vi "PH_SHS_Analysis_Statistician.PC Set Sample Length.vi"(0 "i ref in":refnum<vi>, 2 "Sample Length":i32, 5 "error IO":errorcluster) -> (14 "i ref out":refnum<vi>, 19 "error out":errorcluster)   [LabVIEW 2014, in "PH_SHS_Analysis_Statistician.lvlib"]
uses:
  PH_SHS_Analysis_Statistician.lvlib
  PH_Common/PH_Common.lvlib
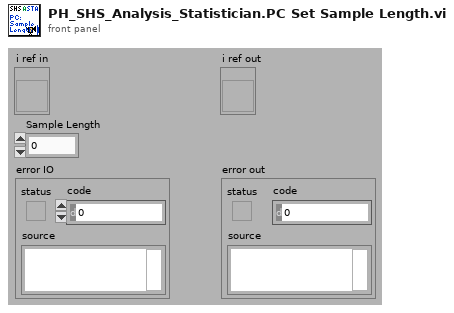
[diagram p1: front panel]
types:
  T1 = typedef "PH_SHS_Analysis_Statistician.lvlib/PH_SHS_Analysis_Statistician.i attribute.ctl" = cluster{"GUI Refs ":cluster{"Status":refnum<vi>, "Result Graph":refnum<vi>, "Mean Data 1":refnum<vi>, "Std Dev Data 1":refnum<vi>, "Mean Data 2":refnum<vi>, "Std Dev Data 2":refnum<vi>, "Mean Data 3":refnum<vi>, "Std Dev Data 3":refnum<vi>, "Dummy Mean":refnum<vi>, "Dummy Std Dev":refnum<vi>, "Export Data":refnum<vi>, "Data 1":refnum<vi>, "Data 2":refnum<vi>, "Data 3":refnum<vi>, "Stat or Trend":refnum<vi>, "Delete":refnum<vi>, "Analyzer":refnum<vi>, "Current Zernike Coefficients":refnum<vi>, "PtV [Lambda]":refnum<vi>, "sample length":refnum<vi>}, "Analyzer":string, "Stat or Trend":bool, "Data 1":i16, "Data 2":i16, "Data 3":i16, "Data":T2[], "sample length":i32, "Datasets strored":i32, "Dataarray Size":i32}
  T2 = typedef "PH_SHS_Analysis.lvlib/PH_SHS_Analysis.Zernike Dataset.ctl" = cluster{"State":T3, "Time Stamp":timestamp, "PtV [lambda]":dbl, "Zernicke Coefficients":T4}
  T3 = typedef "PH_StatusHandler.lvlib/PH_StatusHandler.Status.ctl" = i16
  T4 = typedef "PH_SHS_Analysis.lvlib/PH_SHS_Analysis.Zernike Coefficients.ctl" = cluster{"Tilt x":dbl, "Tilt y":dbl, "Defocus":dbl, "Astig 0°":dbl, "Astig 45°":dbl, "Coma x":dbl, "Coma y":dbl, "Spherical":dbl, "Trefoil 0°":dbl, "Trefoil 30°":dbl, "2nd Astig 0°":dbl, "2nd Astig 45°":dbl, "2nd Coma x":dbl, "2nd Coma y":dbl, "2nd Spherical":dbl}
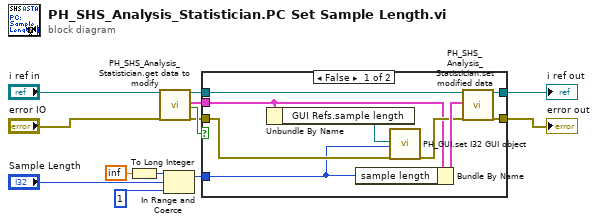
[diagram p0: block diagram]
diagram:
  n1 = To Long Integer(number=inf) -> (32bit integer=w2:i32)
  n2 = call "PH_SHS_Analysis_Statistician.get data to modify.vi"("i ref in"="i ref in", "error in (no error)"="error IO") -> ("i ref out"=w7:refnum<vi>, "i attribute"=w12:T1, "timed out"=w11:bool, "error out"=w9:errorcluster)  [unwired: 14 in]
  n3 = In Range and Coerce(upper limit=w2, x="Sample Length", lower limit=1) -> (coerced(x)=w4:i32)  [unwired: 1 out]
  n4 = case shown="False" w11 {
    tunnel: w7 -> [w22 w24]
    tunnel: [w21 w24] -> w8
    tunnel: w9 -> [w20 w23]
    tunnel: [w19 w23] -> w10
    tunnel: w12 -> [w15 _]
    tunnel: w4 -> [w16 _]
    frame False {
      n5 = Unbundle By Name(w15) -> ("GUI Refs.sample length"=w14:refnum<vi>)
      n6 = Bundle By Name(cluster=w15, "sample length"=w16) -> (w18:T1)
      n7 = call "PH_GUI.set I32 GUI object.vi"("I32 GUI Ref"=w14, "value"=w16, "error in (no error)"=w20) -> ("error out"=w17:errorcluster)  [unwired: 16 in]
      n8 = call "PH_SHS_Analysis_Statistician.set modified data.vi"("i ref in"=w22, "i attribute"=w18, "error in (no error)"=w17) -> ("i ref out"=w21:refnum<vi>, "error out"=w19:errorcluster)  [unwired: 15 in]
    }
    frame True {
    }
  }
  "error out" <- w10
  "i ref out" <- w8
